vi "Client.vi"() -> ()   [LabVIEW 2021, in "Server_Stream.lvlib"]
uses:
  Server_Stream.lvlib
  <vilib>/gRPC/LabVIEW gRPC Library/Shared/grpcId.ctl
  Stream_client/RPC Messages/Acquisition_Control_Stream.ctl
  Stream_client/Stream_client.lvlib
  <vilib>/gRPC/LabVIEW gRPC Library/grpc-lvsupport-release.lvlib
panel:
  in  "Client Address":string="localhost:50051"
  in  "Capture_Count":i32=100
  in  "Start_Capture":bool
  out "Waveform Chart":i32(graph)
  # "Server Stream Client"
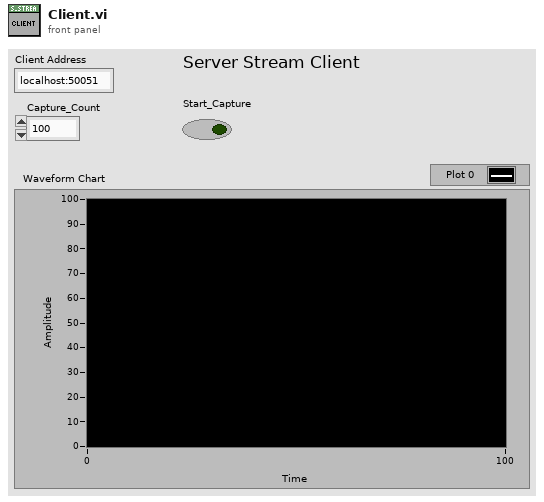
[diagram p1: front panel]
types:
  T1 = typedef "grpc-lvsupport-release.lvlib/grpcId.ctl" = u64
  T2 = cluster{"Call_ID":T1, "Running?":bool, "Stream_Started?":bool}
  T3 = typedef "Stream_client.lvlib/Acquisition_Stream_Data.ctl" = cluster{"Data":i32, "Status":bool}
  T4 = typedef "Stream_client.lvlib/Acquisition_Control_Stream.ctl" = cluster{"Count":i32}
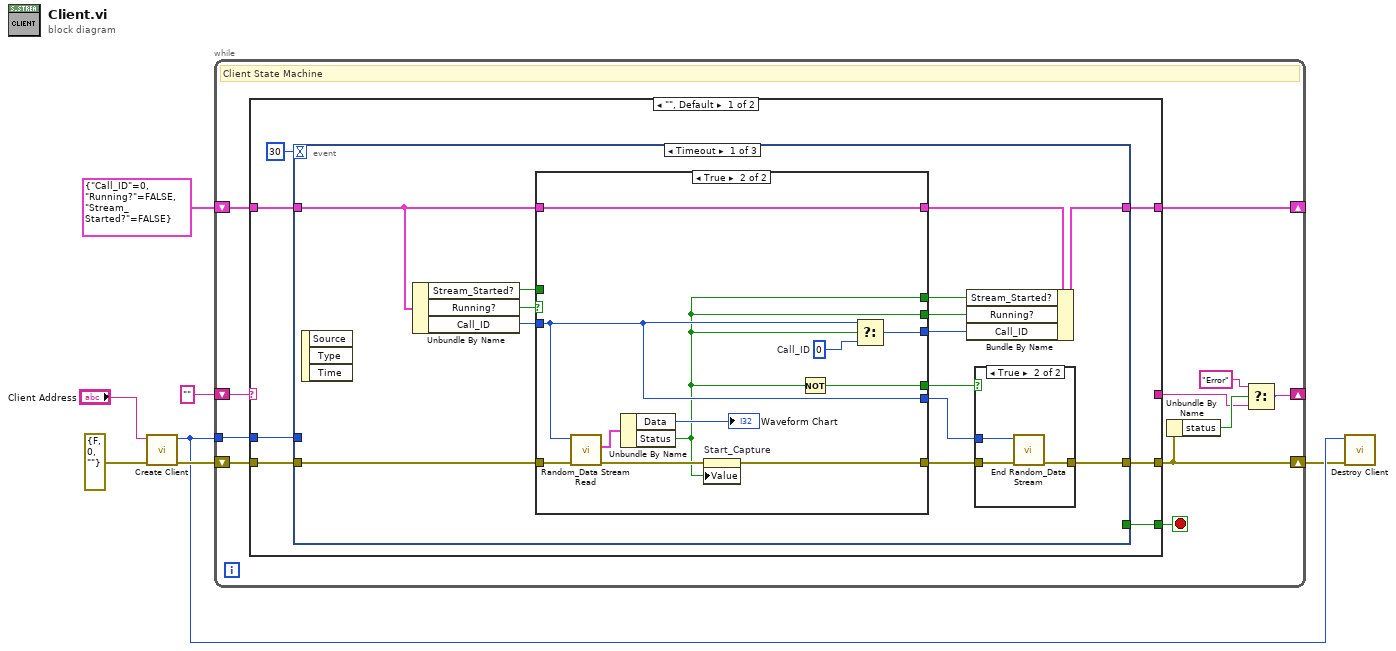
[diagram p0: block diagram]
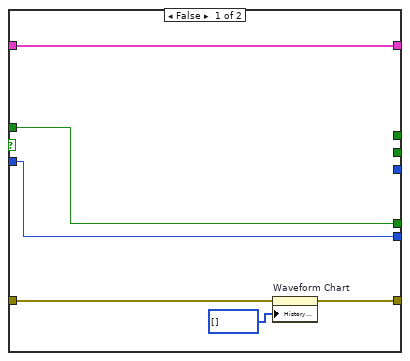
[diagram p3: hidden frame]
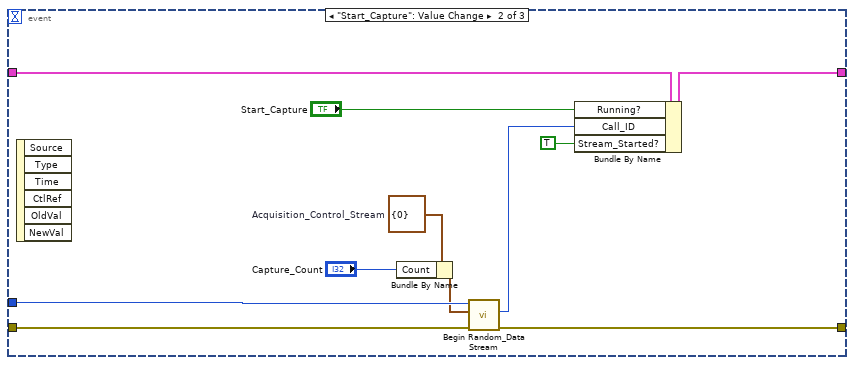
[diagram p4: hidden frame]
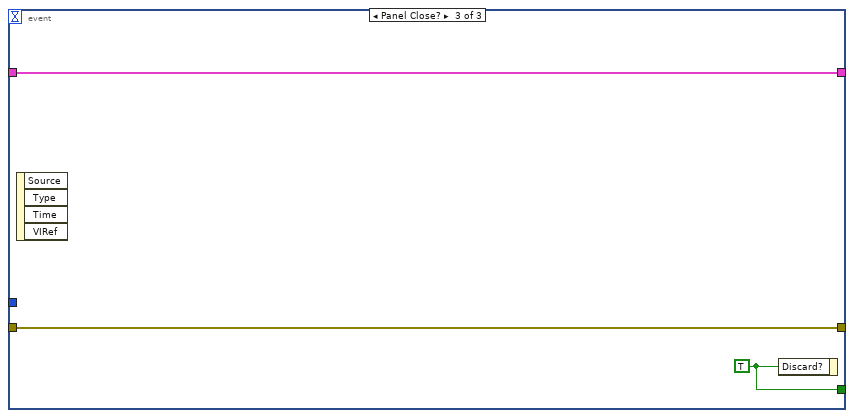
[diagram p5: hidden frame]
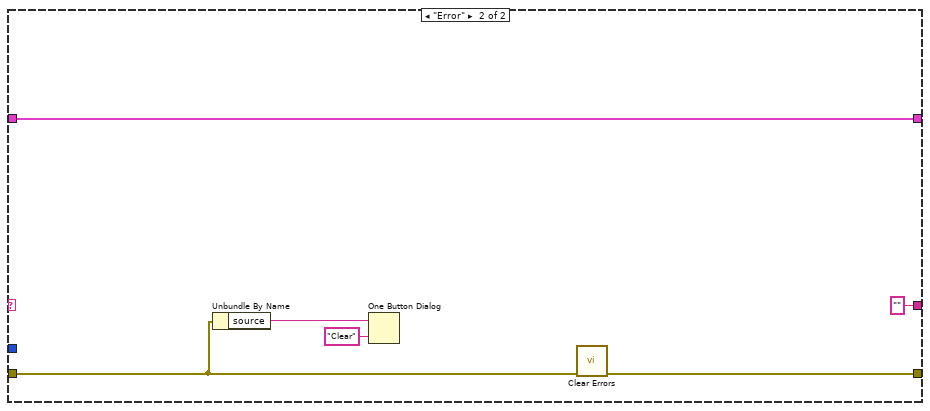
[diagram p6: hidden frame]
diagram:
  n1 = call "Create Client.vi"("error in"=errorcluster {"status"=FALSE, "code"=0, "source"=""} ("error in (no error)"), "address"="Client Address") -> ("error out"=w6:errorcluster, "gRPC ID Out"=w4:T1)  [unwired: 8 in]
  n2 = while {
    shift-right: [w14] -> w2
    shift-left: w6 -> [w17]
    tunnel: w4 -> [w16]
    shift-right: [w12] -> _
    shift-left: "" -> [w18]
    shift-right: [w8] -> _
    shift-left: T2 {"Call_ID"=0, "Running?"=FALSE, "Stream_Started?"=FALSE} -> [w9]
    stop <- w15 stop-if-true
    # "Client State Machine"
    n3 = case shown="\"\", Default" w18 {
      tunnel: w17 -> [w25 w79]
      tunnel: [w24 w80] -> w14
      tunnel: w16 -> [w23 _]
      tunnel: [_ ""] -> w11
      tunnel: [w22 _] -> w15
      tunnel: w9 -> [w20 w75]
      tunnel: [w19 w75] -> w8
      frame "", Default {
        n4 = event shown="[0] Timeout" {
          selector: _ -> [_ _ _]
          dyn-events: _ -> [_ _ _]
          timeout: 30 -> [_ _ _]
          tunnel: w25 -> [w39 w70 w74]
          tunnel: [w30 w63 w74] -> w24
          tunnel: w23 -> [_ w71 _]
          tunnel: [_ _ w73] -> w22
          tunnel: w20 -> [w37 w68 w72]
          tunnel: [w34 w69 w72] -> w19
          event Timeout {
            n5 = event-data() -> ()  [unwired: 1 in, 3 out]
            n6 = Unbundle By Name(w37) -> ("Stream_Started?"=w32:bool, "Running?"=w36:bool, "Call_ID"=w35:T1)
            n7 = case shown="True" w36 {
              tunnel: [w45 w52] -> w29
              tunnel: w39 -> [w44 w59]
              tunnel: w37 -> [w49 w60]
              tunnel: [w49 w60] -> w38
              tunnel: w35 -> [w47 w56]
              tunnel: [_ w50] -> w33
              tunnel: w32 -> [w48 _]
              tunnel: [_ w50] -> w31
              tunnel: [w48 w54] -> w26
              tunnel: [w47 w56] -> w28
              tunnel: [_ w57] -> w27
              frame False {
                n8 = property on="Waveform Chart" class="WFChart (strict)"(error in=w44, "History Data"=i32[] []) -> (error out=w45:errorcluster)  [unwired: 1 in, 1 out]
              }
              frame True {
                w55 = T1 0  # Call_ID
                n9 = call "Random_Data Stream Read.vi"("error in"=w59, "Call ID in"=w56) -> ("error out"=w51:errorcluster, "Response Data"=w58:T3)  [unwired: 6 in, 2 out]
                n10 = Unbundle By Name(w58) -> ("Data"=→"Waveform Chart":i32, "Status"=w50:bool)
                n11 = property on="Start_Capture" class="Bool (strict)"(error in=w51, "Value"=w50) -> (error out=w52:errorcluster)  [unwired: 1 in, 1 out]
                n12 = Not(x=w50) -> (.not. x?=w54:bool)
                n13 = Select(t=w56, s=w50, f=w55) -> (s? t:f=w57:T1)
              }
            }
            n14 = Bundle By Name(cluster=w38, "Stream_Started?"=w31, "Running?"=w33, "Call_ID"=w27) -> (w34:T2)
            n15 = case shown="True" w26 {
              tunnel: [w40 w41] -> w30
              tunnel: w29 -> [w40 w43]
              tunnel: w28 -> [_ w42]
              frame False {
              }
              frame True {
                n16 = call "End Random_Data Stream.vi"("error in"=w43, "Call ID in"=w42) -> ("error out"=w41:errorcluster)  [unwired: 8 in, 1 out]
              }
            }
          }
          event "Start_Capture": Value Change {
            w61 = T4 {"Count"=0}  # Acquisition_Control_Stream
            n17 = event-data() -> ()  [unwired: 1 in, 6 out]
            n18 = Bundle By Name(cluster=w61, "Count"="Capture_Count") -> (w65:T4)
            n19 = call "Begin Random_Data Stream.vi"("error in"=w70, "Request Data"=w65, "gRPC ID"=w71) -> ("error out"=w63:errorcluster, "Call Id Out"=w67:T1)  [unwired: 6 in, 1 out]
            n20 = Bundle By Name(cluster=w68, "Running?"="Start_Capture", "Call_ID"=w67, "Stream_Started?"=TRUE ("Stream Used?")) -> (w69:T2)
          }
          event Panel Close? {
            w73 = TRUE ("Discard?")
            n21 = event-data() -> ()  [unwired: 1 in, 4 out]
            n22 = event-data("Discard?"=w73) -> ()  [unwired: 1 in, 1 out]
          }
        }
      }
      frame "Error" {
        n23 = Unbundle By Name(w79) -> ("source"=w77:string)
        n24 = One Button Dialog(message=w77, button name ("OK")="Clear") -> ()  [unwired: 1 out]
        n25 = call <vilib>:"Clear Errors.vi"("error in (no error)"=w79) -> ("error out"=w80:errorcluster)  [unwired: 5 in, 1 out]
      }
    }
    n26 = Unbundle By Name(w14) -> ("status"=w13:bool)
    n27 = Select(t="Error", s=w13, f=w11) -> (s? t:f=w12:string)
  }
  n28 = call "Destroy Client.vi"("error in"=w2, "gRPC ID"=w4) -> ()  [unwired: 9 in, 1 out]
